vi "FGV_Multipositions_Array.vi"(8 "error in":errorcluster, 10 "Action":T1, 11 "Multipositions array IN":dbl[][](array[numeric])) -> (0 "error out":errorcluster, 2 "Multiposition Size":u16, 3 "Multipositions array OUT":dbl[][](array[numeric]))   [LabVIEW 2026]
doc: "Functional Global Variable:\n- Write the value into the memory \nor\n- Read the value from the memory"
uses:
  TypeDef_FGV.ctl
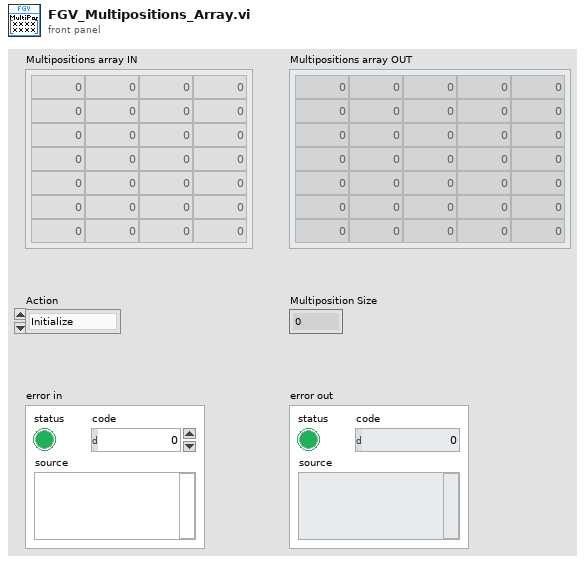
[diagram p1: front panel]
types:
  T1 = typedef "TypeDef_FGV.ctl" = enum16{"Initialize", "Write", "Read", "Read_File", "Write_to_File"}
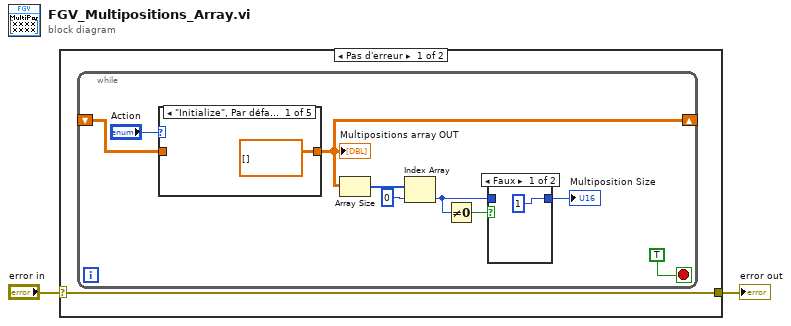
[diagram p0: block diagram]
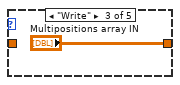
[diagram p4: hidden frame]
diagram:
  n1 = case shown="Pas d'erreur" "error in" {
    selector: "error in" -> [w3 w20]
    tunnel: [w3 w20] -> w1
    frame No Error {
      n2 = while {
        shift-right: [w7] -> _
        shift-left: _ -> [w10]
        stop <- TRUE stop-if-true
        n3 = case shown="\"Initialize\", Par défaut" "Action" {
          tunnel: w10 -> [_ w16 _ w18 w19]
          tunnel: [dbl[][] [] w16 "Multipositions array IN" w18 w19] -> w7
          frame "Initialize", Default {
          }
          frame "Read" {
          }
          frame "Write" {
          }
          frame "Read_File" {
            # "A FAIRE"
          }
          frame "Write_to_File" {
            # "A Faire"
          }
        }
        "Multipositions array OUT" <- w7
        n4 = Array Size(array=w7) -> (size(s)=w9:i32[])
        n5 = Index Array(array=w9, index=u8 0) -> (element=w4:i32)
        n6 = Not Equal To 0?(x=w4) -> (x != 0?=w6:bool)
        n7 = case shown="Faux" w6 {
          tunnel: [1 w14] -> w5
          tunnel: w4 -> [_ w14]
          frame False {
          }
          frame True {
          }
        }
        "Multiposition Size" <- w5
      }
    }
    frame Error {
    }
  }
  "error out" <- w1
